vi "Climber Controller.vi"(8 "error in":errorcluster) -> ()   [LabVIEW 2019]
doc: "This VI executes continuously carrying out the current operation and responding to updates or new operations. It will often contain the timing or control code that is difficult to place directly in TeleOp. This VI generally opens all sensors and motors and isolates the rest of the robot code from knowing how the operations are carried out."
uses:
  Climber Operations.ctl
  Climber Setpoints.ctl
  <vilib>/Rock Robotics/WPI/SafetyOutput/WPI_SafetyOutputConfigMenu.ctl
  <vilib>/Rock Robotics/WPI/Solenoid/WPI_SolenoidChannel.ctl
  <vilib>/Rock Robotics/Network Tables/NT Write Boolean.vi
  <vilib>/Rock Robotics/WPI/Solenoid/WPI_SolenoidSetEnum.vi
  <vilib>/Rock Robotics/WPI/Solenoid/WPI_SolenoidGetEnum.vi
  <vilib>/Rock Robotics/WPI/Solenoid/WPI_SolenoidOpenSingle.vi
  <vilib>/Rock Robotics/WPI/Solenoid/WPI_SolenoidValue.ctl
  <vilib>/Rock Robotics/WPI/Framework/Completion Status.ctl
panel:
  out "Value 2":T1
  in  "Interactive Values":T2
  out "Current\nCmd":string
  in  "Buttons":cluster{"Execute Cmd":bool, "Abort Cmd":bool}
  out "Command Timing":cluster{"Start Time (ms)":u32, "Iterations":i32}
  out "Status":T4
  # "Tip: It may be helpful to observe inputs and sensor values.\nYou may also want to display tuning or debugging controls."
  # "Interactive Command: You may fill in the settings for a command\nand schedule it with the Execute button. You can observe and abort\nany command while fine tuning the code for the controller."
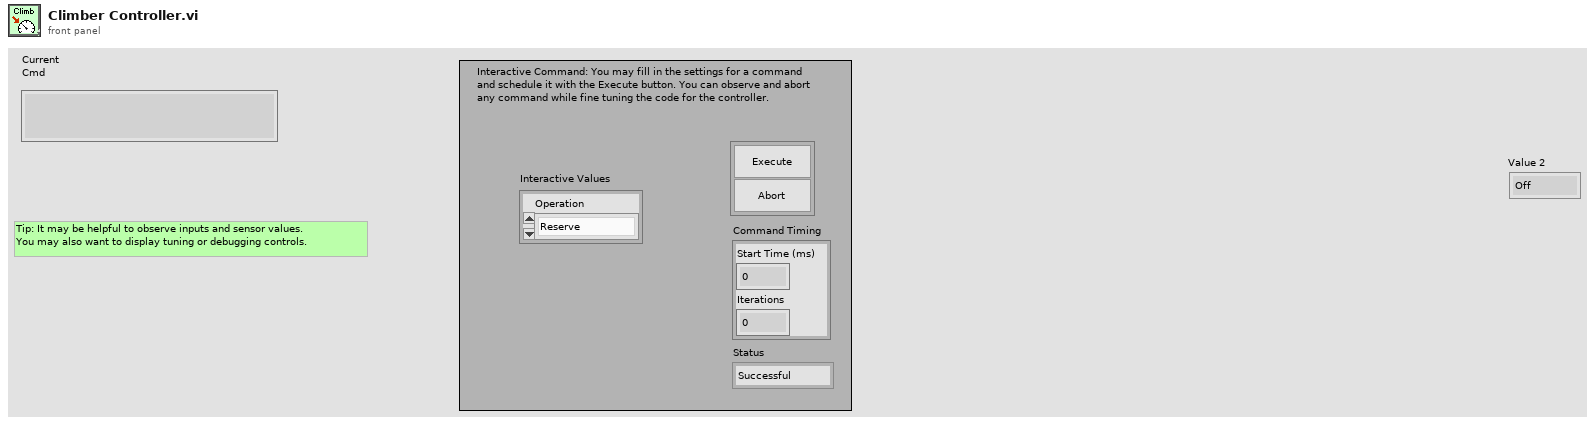
[diagram p1: front panel]
types:
  T1 = typedef "WPI_SolenoidValue.ctl" = enum16{"Off", "On", "Forward", "Reverse"}
  T2 = typedef "Climber Setpoints.ctl" = cluster{"Operation":T3}
  T3 = typedef "Climber Operations.ctl" = enum16{"Reserve", "Read Current", "Immediate", "Climb Raise", "Climb Lower"}
  T4 = typedef "Completion Status.ctl" = enum16{"Successful", "Aborted", "Incomplete"}
  T5 = typedef "WPI_SolenoidChannel.ctl" = enum8{"Solenoid 0", "Solenoid 1", "Solenoid 2", "Solenoid 3", "Solenoid 4", "Solenoid 5", "Solenoid 6", "Solenoid 7", "Invalid"}
  T6 = typedef "WPI_SafetyOutputConfigMenu.ctl" = enum16{"Enable", "Disable"}
  T7 = typedef "WPI_SolenoidDevRef.ctl" = cluster{"DevStatus":errorcluster, "Pneumatics Control Module":u8, "Forward Solenoid Channel":T5, "Reverse Solenoid Channel":T5}
  T8 = typedef "Command Status Info.ctl" = cluster{"Name":string, "Status":T4, "notifier out":T9}
  T9 = typedef "Completion Notifier.ctl" = refnum<notifier>
  T10 = cluster{"Current Command":T2, "Command Timing":cluster{"Start Time (ms)":u32, "Iterations":i32}, "Command Arguments":cluster{"Command Info":T8, "Description":string, "Default Command":T2, "queue out":refnum<queue>, "Subsystem Name":string}}
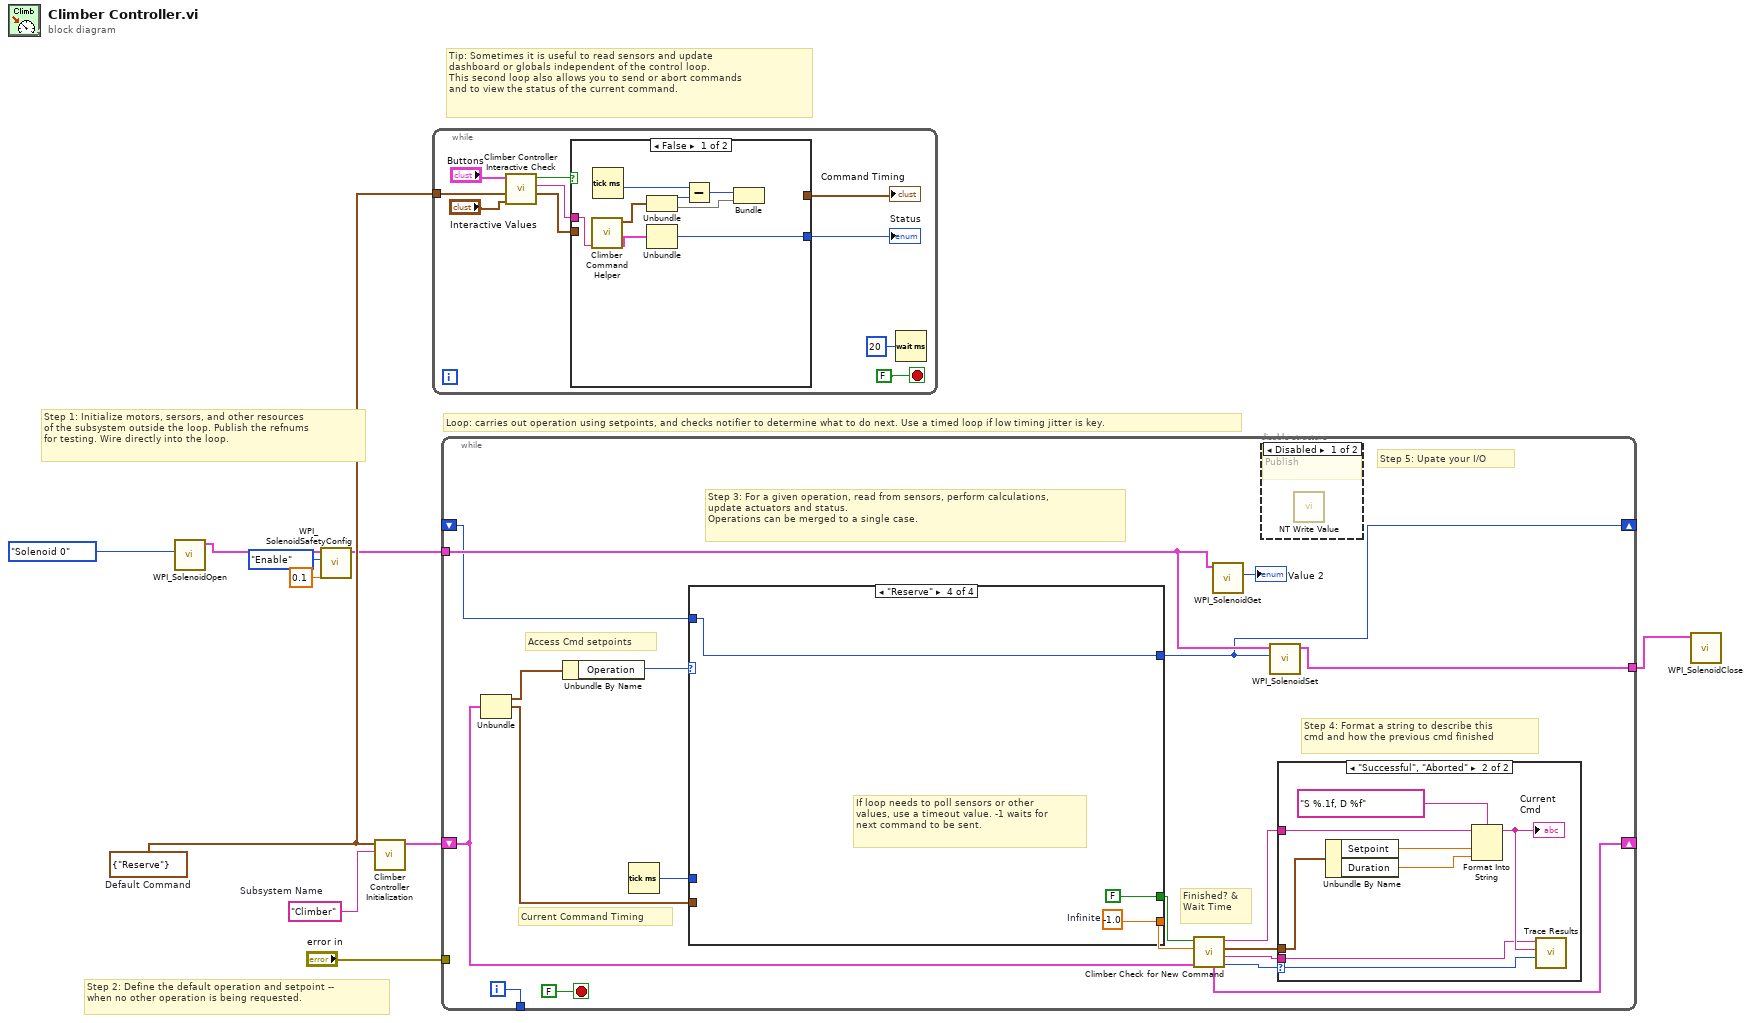
[diagram p0: block diagram]
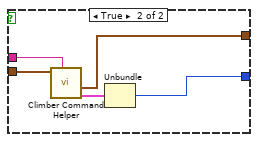
[diagram p2: hidden frame]
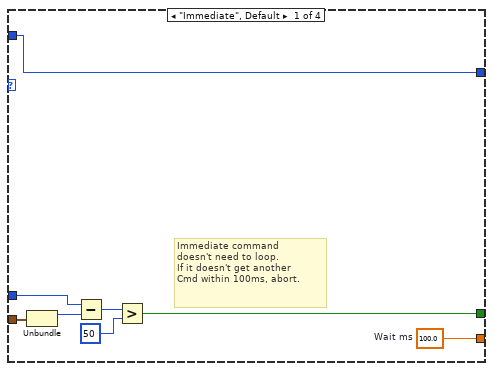
[diagram p5: hidden frame]
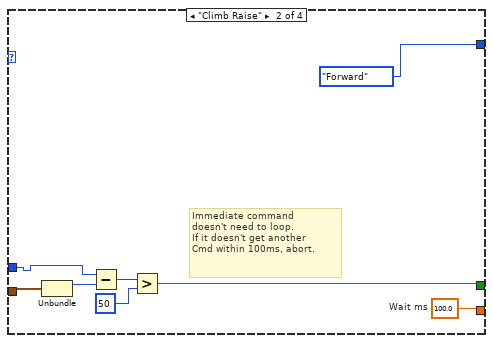
[diagram p6: hidden frame]
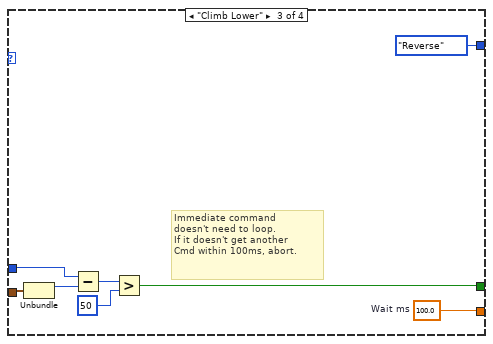
[diagram p7: hidden frame]
diagram:
  w7 = T2 {"Operation"=enum."Reserve"}  # Default Command
  w8 = "Climber"  # Subsystem Name
  # "Tip: Sometimes it is useful to read sensors and update\ndashboard or globals independent of the control loop.\nThis second loop also allows you to send or abort commands\nand to view the status of the current command."
  # "Step 2: Define the default operation and setpoint --\nwhen no other operation is being requested."
  # "Step 1: Initialize motors, sersors, and other resources\nof the subsystem outside the loop. Publish the refnums\nfor testing. Wire directly into the loop."
  # "Loop: carries out operation using setpoints, and checks notifier to determine what to do next. Use a timed loop if low timing jitter is key."
  n1 = call-poly <vilib>:"WPI_SolenoidOpen.vi"("Solenoid Channel"=WPI_SolenoidChannel."Solenoid 0") -> ("SolenoidDevRef"=w6:T7)  [unwired: 9 in, 1 out]
  n2 = call <vilib>:"WPI_SolenoidSafetyConfig.vi"("timeout (s)"=0.1, "mode"=WPI_SafetyOutputConfigMenu."Enable", "SolenoidDevRef"=w6) -> ("SolenoidDevRef"=w1:T7)  [unwired: 7 in, 1 out]
  n3 = call "Climber Controller Initialization.vi"("Subsystem Name"=w8, "Default Command"=w7) -> ("Current Command"=w9:T10)  [unwired: 9 in]
  n4 = while {
    tunnel: w7 -> [w17]
    stop <- FALSE stop-if-true
    n5 = call "Climber Controller Interactive Check.vi"("Interactive Command in"="Interactive Values", "Default Command"=w17, "Buttons"="Buttons") -> ("Interactive Command out"=w14:T2, "Trace String"=w15:string, "Schedule"=w16:bool)  [unwired: 6 in]
    n6 = case shown="False" w16 {
      tunnel: [w28 w33] -> w13
      tunnel: w14 -> [_ w31]
      tunnel: [_ w29] -> w12
      tunnel: w15 -> [w21 w32]
      frame False {
        n7 = call "Climber Command Helper.vi"("Command Info In"=w21) -> ("Command Info Out"=w23:T8, "SubSystem Data"=w22:T2)  [unwired: 8 in, 1 out]
        n8 = Tick Count (ms)() -> (millisecond timer value=w24:u32)
        n9 = Unbundle(w22) -> (w27:T3, w25)
        n10 = Unbundle(w23) -> ("Status"=w28:T4)  [unwired: 2 out]
        n11 = Subtract(x=w24, y=w27) -> (x-y=w26:u32)
        n12 = Bundle(w26, w25) -> ()  [unwired: 1 in, 1 out]
      }
      frame True {
        n13 = call "Climber Command Helper.vi"("Description"=w32, "SubSystem Data"=w31) -> ("Command Info Out"=w30:T8, "Command Timing"=w29:cluster{"Start Time (ms)":u32, "Iterations":i32})  [unwired: 7 in, 1 out]
        n14 = Unbundle(w30) -> ("Status"=w33:T4)  [unwired: 2 out]
      }
    }
    "Status" <- w13
    "Command Timing" <- w12
    n15 = Wait (ms)(milliseconds to wait=u32 20) -> ()  [unwired: 1 out]
  }
  n16 = while {
    shift-right: [w46] -> _
    shift-left: w9 -> [w39]
    tunnel: [w51] -> _
    tunnel: "error in" -> [_]
    tunnel: [w37] -> w2
    tunnel: w1 -> [w36]
    shift-right: [w35] -> _
    shift-left: _ -> [w34]
    i -> [w51]
    stop <- FALSE stop-if-true
    # "Step 5: Upate your I/O"
    # "Step 4: Format a string to describe this\ncmd and how the previous cmd finished"
    # "Current Command Timing"
    # "Access Cmd setpoints"
    # "Finished? &\nWait Time"
    # "Step 3: For a given operation, read from sensors, perform calculations,\nupdate actuators and status.\nOperations can be merged to a single case."
    n17 = Unbundle(w39) -> ("Current Command"=w50:T2, "Command Timing"=w47:cluster{"Start Time (ms)":u32, "Iterations":i32})  [unwired: 1 out]
    n18 = Unbundle By Name(w50) -> ("Operation"=w49:T3)
    n19 = Tick Count (ms)() -> (millisecond timer value=w48:u32)
    n20 = case shown="\"Reserve\"" w49 {
      tunnel: [w68 w72 w80 w87] -> w44
      tunnel: [w62 w73 w81 FALSE ("ignore previous (F)")] -> w45
      tunnel: w47 -> [w64 w70 w78 _]
      tunnel: w48 -> [w63 w71 w79 _]
      tunnel: [w61 WPI_SolenoidValue."Forward" ("Value") WPI_SolenoidValue."Reverse" ("Value") w85] -> w35
      tunnel: w34 -> [w61 _ _ w85]
      frame "Immediate", Default {
        w68 = 100.0  # Wait ms
        # "Immediate command\ndoesn't need to loop.\nIf it doesn't get another\nCmd within 100ms, abort."
        n21 = Unbundle(w64) -> ("Start Time (ms)"=w67:u32)  [unwired: 1 out]
        n22 = Subtract(x=w63, y=w67) -> (x-y=w66:u32)
        n23 = Greater?(x=w66, y=u8 50 ("Left Motor")) -> (0:w62:bool)
      }
      frame "Climb Raise" {
        w72 = 100.0  # Wait ms
        # "Immediate command\ndoesn't need to loop.\nIf it doesn't get another\nCmd within 100ms, abort."
        n24 = Unbundle(w70) -> ("Start Time (ms)"=w76:u32)  [unwired: 1 out]
        n25 = Subtract(x=w71, y=w76) -> (x-y=w75:u32)
        n26 = Greater?(x=w75, y=u8 50 ("Left Motor")) -> (0:w73:bool)
      }
      frame "Climb Lower" {
        w80 = 100.0  # Wait ms
        # "Immediate command\ndoesn't need to loop.\nIf it doesn't get another\nCmd within 100ms, abort."
        n27 = Unbundle(w78) -> ("Start Time (ms)"=w84:u32)  [unwired: 1 out]
        n28 = Subtract(x=w79, y=w84) -> (x-y=w83:u32)
        n29 = Greater?(x=w83, y=u8 50 ("Left Motor")) -> (0:w81:bool)
      }
      frame "Reserve" {
        w87 = -1.0  # Infinite
        # "If loop needs to poll sensors or other\nvalues, use a timeout value. -1 waits for\nnext command to be sent."
      }
    }
    n30 = call "Climber Check for New Command.vi"("Current Command"=w39, "Wait time (ms)"=w44, "Finished?"=w45) -> ("Completion"=w40:T4, "Subsystem Name"=w41:string, "Current Command"=w42:T2, "Initial Trace String"=w43:string, "NextCommand"=w46:T10)  [unwired: 4 in]
    n31 = call-poly <vilib>:"WPI_SolenoidGet.vi"("SolenoidDevRef"=w36) -> ("Value"=→"Value 2":T1)  [unwired: 8 in, 2 out]
    n32 = disable-structure shown="Disabled" {
      frame Disabled {
        # "Publish"
        n33 = call-poly <vilib>:"NT Write Value.vi"() -> ()  [unwired: 11 in, 1 out]
      }
      frame Enabled {
      }
    }
    n34 = call-poly <vilib>:"WPI_SolenoidSet.vi"("Value"=w35, "SolenoidDevRef"=w36) -> ("SolenoidDevRef"=w37:T7)  [unwired: 8 in, 1 out]
    n35 = case shown="\"Successful\", \"Aborted\"" w40 {
      selector: w40 -> [_ w60]
      tunnel: w43 -> [_ w56]
      tunnel: w42 -> [_ w57]
      tunnel: w41 -> [_ w53]
      frame "Incomplete", Default {
        # "Continuing current command"
      }
      frame "Successful", "Aborted" {
        # "Report and setup for next command"
        n36 = Unbundle By Name(w57) -> ("Setpoint"=w59:dbl, "Duration"=w54:dbl)
        n37 = Format Into String(format string="S %.1f, D %f", initial string=w56, w59, w54) -> (resulting string=w55:string)  [unwired: 1 in, 1 out]
        "Current\nCmd" <- w55
        n38 = call <vilib>:"Trace Results.vi"("Status of previous command"=w60, "Description"=w55, "Subsystem"=w53) -> ()  [unwired: 9 in]
      }
    }
  }
  n39 = call <vilib>:"WPI_SolenoidClose.vi"("SolenoidDevRef"=w2) -> ()  [unwired: 10 in, 1 out]
